vi "Ophir EnergyFlag.vi"(0 "Visa Session":refnum<visa-resource-name>, 1 "error in (no error)":errorcluster) -> (2 "dup Visa Session":refnum<visa-resource-name>, 3 "Energy Flag?":bool, 4 "error out":errorcluster)   [LabVIEW 2017]
doc: "EnergyFlag.vi checks if instrument has measured a new energy pulse\nVersion 2.00\nLast Updated 16 March 2005\n\nInputs\nVisa Session\nErrorIn\nOutputs\ndup Visa Session\nEnergy Flag? True if instrument has measured a new energy pulse\nErrorOut\nReturns Error n# -1328 when Energy Flag Failed"
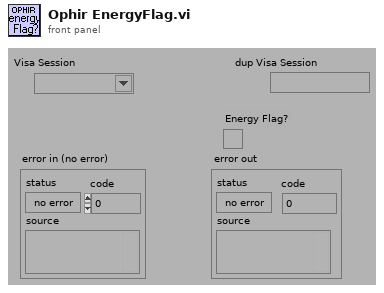
[diagram p1: front panel]
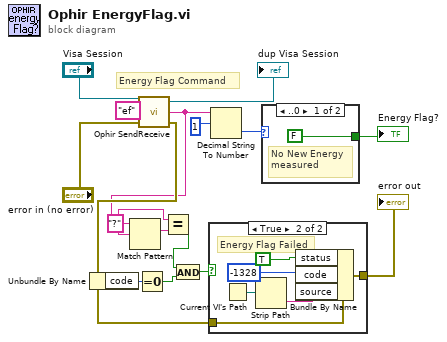
[diagram p0: block diagram]
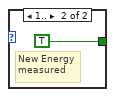
[diagram p3: hidden frame]
diagram:
  w7 = "?"
  # "Energy Flag Command"
  n1 = call "Ophir SendReceive.vi"("error in (no error)"="error in (no error)", "Command"="ef", "Visa Session"="Visa Session") -> ("error out"=w3:errorcluster, "Frame Output"=w2:string, "dup Visa Session"=→"dup Visa Session":refnum<visa-resource-name>)
  n2 = Unbundle By Name(w3) -> ("code"=w9:i32)
  n3 = Match Pattern(string=w2, regular expression=w7) -> (match substring=w6:string)  [unwired: 4 out]
  n4 = Equal To 0?(x=w9) -> (x = 0?=w8:bool)
  n5 = Equal?(x=w7, y=w6) -> (x = y?=w5:bool)
  n6 = And(x=w5, y=w8) -> (x .and. y?=w4:bool)
  n7 = case shown="True" w4 {
    tunnel: w3 -> [w17 w20]
    tunnel: [w17 w19] -> w1
    frame False {
      # "No Error or \nError already exists"
    }
    frame True {
      # "Energy Flag Failed"
      n8 = Current VI's Path() -> (path=w18:path)
      n9 = Strip Path(path=w18) -> (name=w21:string)  [unwired: 1 out]
      n10 = Bundle By Name(cluster=w20, "status"=TRUE, "code"=-1328, "source"=w21) -> (w19:errorcluster)
    }
  }
  "error out" <- w1
  n11 = Decimal String To Number(string=w2, offset=1) -> (number=w11:i32)  [unwired: 2 out]
  n12 = case shown="..0" w11 {
    tunnel: [FALSE TRUE] -> w10
    frame ..0 {
      # "No New Energy\nmeasured"
    }
    frame 1.. {
      # "New Energy\nmeasured"
    }
  }
  "Energy Flag?" <- w10
